vi "main_ZEST.vi"() -> ()   [LabVIEW 2022 SP3]
uses:
  <vilib>/Analysis/1siggen.llb/Ramp Pattern by Samples.vi
  <vilib>/Analysis/NI_AALBase.lvlib
panel:
  out "likehood function":cluster{"Ramp Pattern":dbl[], "y":dbl[]}(graph)
  out "q(i)":cluster{"Ramp Pattern":dbl[], "Y":dbl[]}(graph)
  out "Cummulative Threshold Estimate [dB]":dbl=19.38227816273107
  out "Threshold approaching":dbl[][](graph)
  out "initial p.d.f. - q(0)":cluster{"Ramp Pattern":dbl[], "Y":dbl[]}(graph)
  out "psychometric function":cluster{"Ramp Pattern":dbl[], "y":dbl[]}(graph)
  in  "beta":dbl=3.5
  out "T(i) [dB]":dbl=10.0
  in  "T(0) [dB]":dbl=10.0
  in  "sigma":dbl=5.0
  in  "N":i32=4000
  in  "Max power [dB]":dbl=100.0 format="%0.2f"
  in  "Min power [dB]":dbl format="%0.2f"
  # "`"
  # "EXAMPLE; AUDIO SPECTRAL SENSITIVITY"
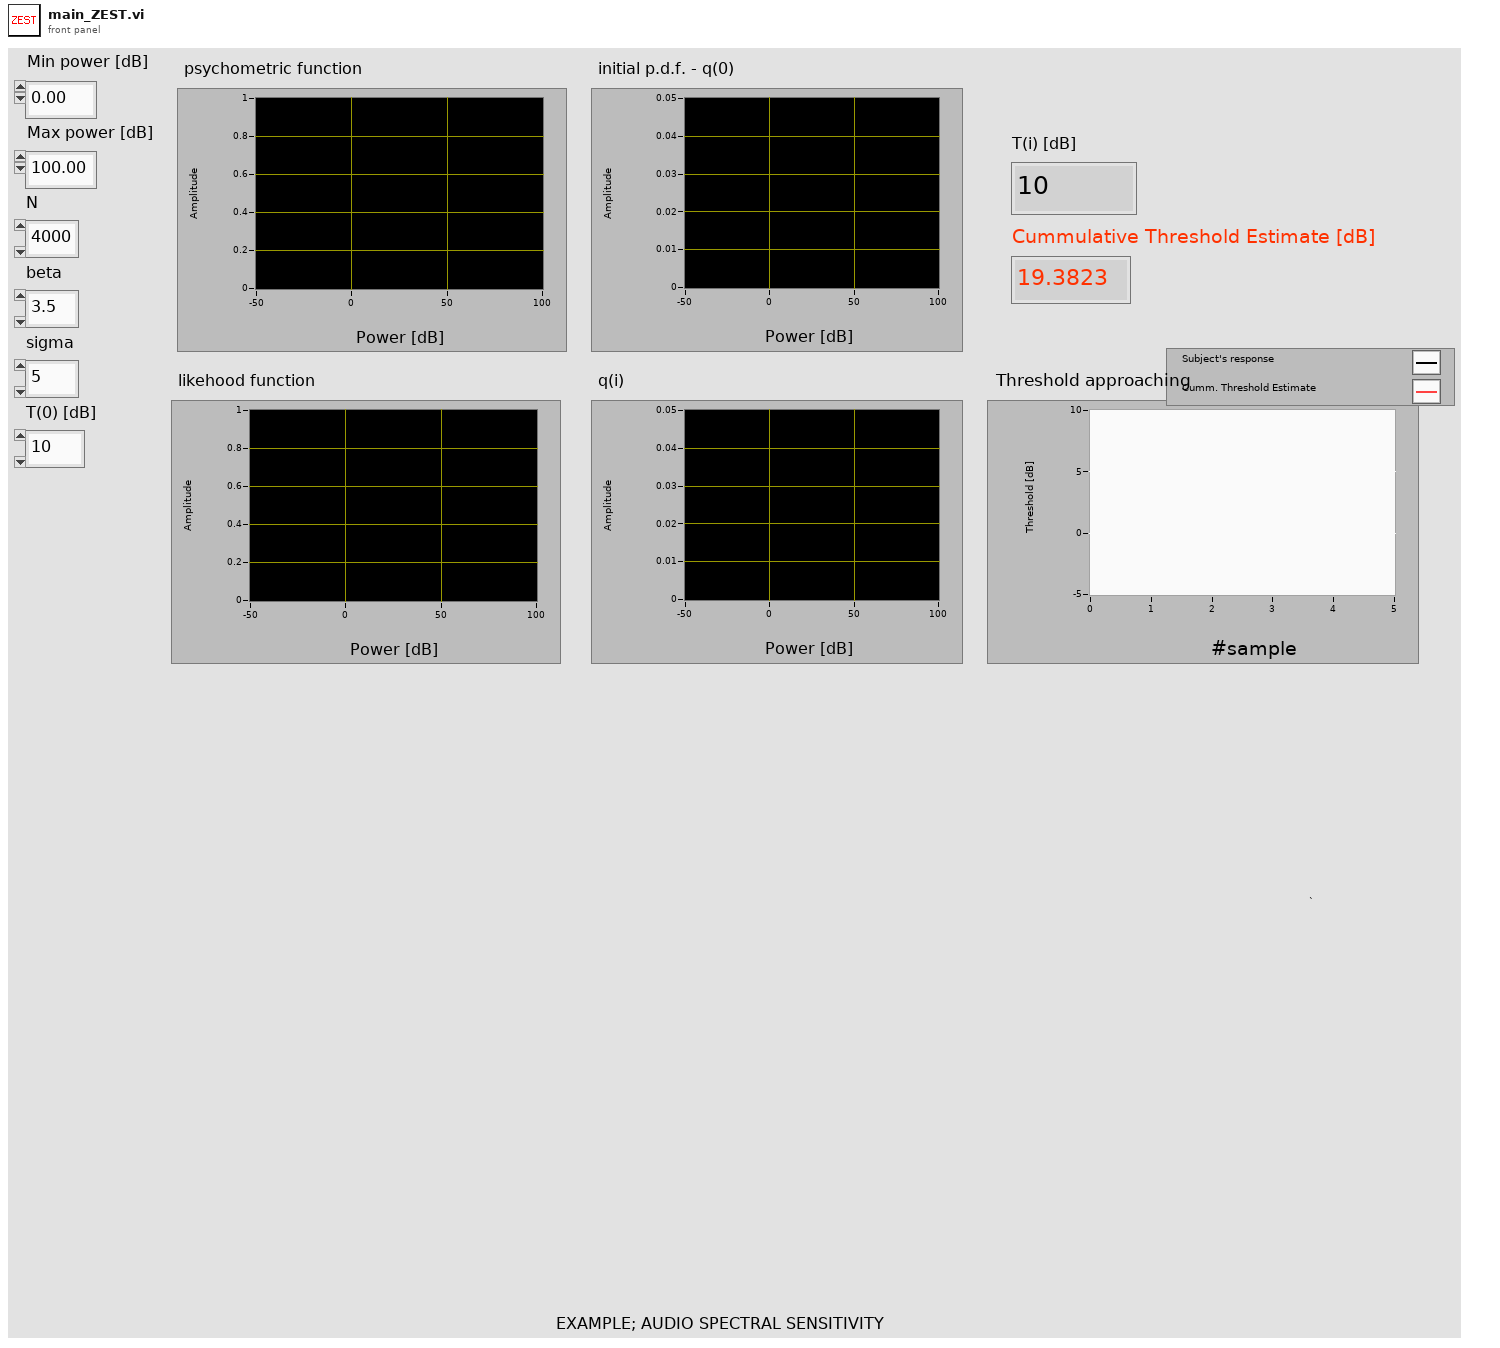
[diagram p1: front panel]
types:
  T1 = typedef "eventvkey.ctl" = enum16{"ASCII", "Enter", "Return", "Shift", "Ctrl", "Alt", "Cmd", "Opt", "Caps", "NumLock", "Clear", "Break", "Up", "Down", "Left", "Right", "Insert", "Delete", "Home", "End", "PageUp", "PageDown", "Escape", "Help", "Pause", "ScrollLock", "F1", "F2", "F3", "F4", "F5", "F6", "F7", "F8", "F9", "F10", "F11", "F12", "F13", "F14", "F15", "F16", "F17", "F18", "F19", "F20", "F21", "F22", "F23", "F24", "Play", "VolumeUp", "VolumeDown", "Mute", "Two Byte Char"}
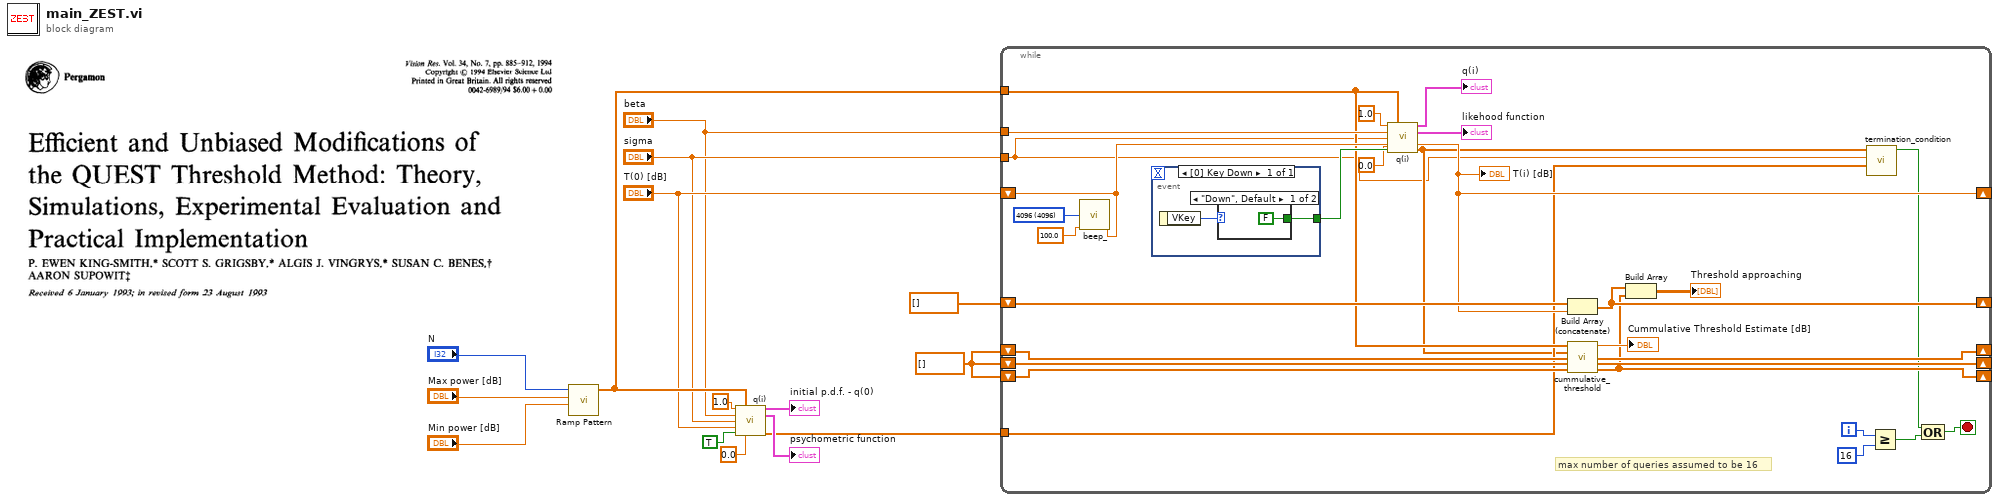
[diagram p0: block diagram]
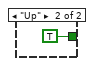
[diagram p2: hidden frame]
diagram:
  w11 = dbl[] []
  n1 = call-poly <vilib>:"Ramp Pattern.vi"("start"="Min power [dB]", "end"="Max power [dB]", "samples"="N") -> ("Ramp Pattern"=w10:dbl[])  [unwired: 7 in, 1 out]
  n2 = call "q(i).vi"("Amplitude"=1.0, "N"=w10, "beta"="beta", "sigma"="sigma", "T(0) [dB]"="T(0) [dB]", "Response"=TRUE, "offset"=0.0) -> (4:"q(i)"=→"initial p.d.f. - q(0)":cluster{"Ramp Pattern":dbl[], "Y":dbl[]}, "likehood function"=→"psychometric function":cluster{"Ramp Pattern":dbl[], "y":dbl[]}, 15:"q(i)"=w1:dbl[])  [unwired: 5 in, 1 out]
  n3 = while {
    tunnel: w10 -> [w29]
    shift-right: [w34] -> _
    shift-left: "T(0) [dB]" -> [w37]
    shift-right: [w32] -> _
    shift-left: dbl[] [] -> [w35]
    shift-right: [w19] -> _
    shift-left: w11 -> [w27]
    shift-right: [w17] -> _
    shift-left: w11 -> [w28]
    shift-right: [w31] -> _
    shift-left: w11 -> [w26]
    tunnel: "beta" -> [w38]
    tunnel: "sigma" -> [w20]
    tunnel: w1 -> [w22]
    i -> [w18]
    stop <- w23 stop-if-true
    w43 = 4096 items=["128"=128, "256 "=256, "500"=512, "1024"=1024, "2048"=2048, "4096"=4096, "8192"=8192, "16384"=16384] ("Duration (au):")
    # "max number of queries assumed to be 16"
    n4 = call "beep_.vi"("Block Size"=w43, "Frequency"=100.0, "volume"=w37) -> ()  [unwired: 12 in, 1 out]
    n5 = event shown="[0] Key Down" {
      selector: _ -> [_]
      dyn-events: _ -> [_]
      timeout: _ -> [_]
      tunnel: [w45] -> w40
      event Key Down {
        n6 = event-data() -> ("VKey"=w46:T1)  [unwired: 1 in]
        n7 = case shown="\"Down\", Default" w46 {
          tunnel: [FALSE ("Sign") TRUE ("Sign")] -> w45
          frame "Down", Default {
          }
          frame "Up" {
          }
        }
      }
    }
    n8 = call "q(i).vi"("Amplitude"=1.0, "N"=w29, "beta"=w38, "sigma"=w20, "T(0) [dB]"=w37, "Response"=w40, "offset"=0.0) -> (4:"q(i)"=→"q(i)":cluster{"Ramp Pattern":dbl[], "Y":dbl[]}, "likehood function"=→"likehood function":cluster{"Ramp Pattern":dbl[], "y":dbl[]}, "T(i)"=w34:dbl, 15:"q(i)"=w21:dbl[])  [unwired: 5 in]
    "T(i) [dB]" <- w34
    n9 = Build Array (concatenate)(w35, w34) -> (w32:dbl[])
    n10 = call "cummulative_threshold.vi"("N"=w29, "q(i)"=w21, "Array 1 in"=w26, "Array 2 in"=w27, "Array 3 in"=w28) -> ("Cummulative Threshold Estimate [dB]"=→"Cummulative Threshold Estimate [dB]":dbl, "Array 1 out"=w31:dbl[], "Array 2 out"=w19:dbl[], "Array 3 out"=w17:dbl[])  [unwired: 7 in]
    n11 = Build Array(w32, w17) -> (→"Threshold approaching":dbl[][])
    n12 = call "termination_condition.vi"("q(0)"=w22, "sigma"=w20, "q(i)"=w21) -> ("Y/N"=w16:bool)  [unwired: 8 in]
    n13 = Greater Or Equal?(x=w18, y=16) -> (x >= y?=w25:bool)
    n14 = Compound Arithmetic op=OR(w16, w25) -> (w23:bool)
  }
